vi "Setup.vi"(11 "jettl Msg Setup in":refnum<class "jettl Msg Setup.lvclass">) -> (3 "jettl Msg Setup out":refnum<class "jettl Msg Setup.lvclass">)   [LabVIEW 2021, in "jettl Msg Setup.lvlib" / "jettl Msg Setup.lvclass"]
uses:
  jettl Msg Setup.lvclass
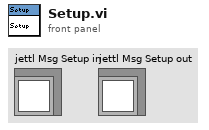
[diagram p1: front panel]
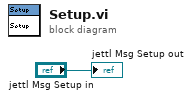
[diagram p0: block diagram]
diagram:
  "jettl Msg Setup out" <- "jettl Msg Setup in"
